vi "Start Acquisition.vi"(8 "error in (no error)":errorcluster, 11 "CCDCamera in":refnum<class "CCDCamera.lvclass">) -> (0 "error out":errorcluster, 3 "CCDCamera out":refnum<class "CCDCamera.lvclass">)   [LabVIEW 2018, in "CCDCamera.lvclass"]
doc: "This VI sends to the camera the command to start acquisition."
uses:
  CCDCamera.lvclass
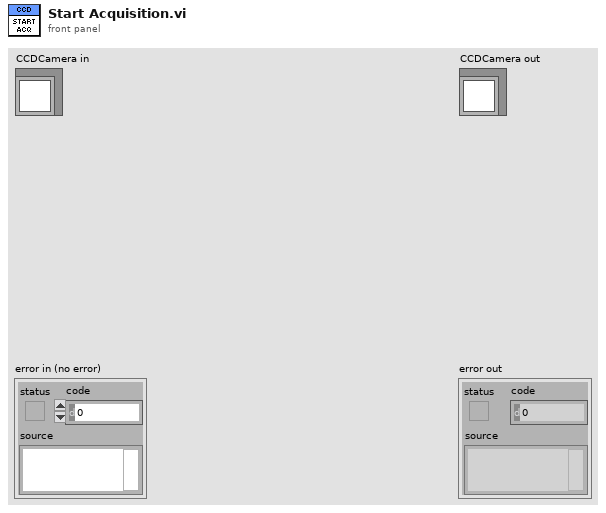
[diagram p1: front panel]
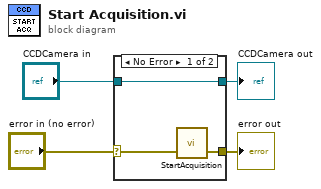
[diagram p0: block diagram]
diagram:
  n1 = case shown="No Error" "error in (no error)" {
    selector: "error in (no error)" -> [w6 w9]
    tunnel: [w7 w9] -> w3
    tunnel: [w5 w8] -> w1
    tunnel: "CCDCamera in" -> [w5 w8]
    frame No Error {
      n2 = call <userlib>:"StartAcquisition.vi"("error in (no error)"=w6) -> ("error out"=w7:errorcluster)  [unwired: 1 in, 1 out]
    }
    frame Error {
    }
  }
  "error out" <- w3
  "CCDCamera out" <- w1
